vi "Data Read Single.vi"(0 "VISA resource name":refnum<visa-resource-name>, 5 "error in (no error)":errorcluster) -> (14 "VISA resource name out":refnum<visa-resource-name>, 15 "Measurement":dbl format="%#_6e", 19 "error out":errorcluster)   [LabVIEW 2024, in "Keithley 2100 Series.lvlib"]
doc: "This VI reads a measurement or calculation from the instrument. It also returns the channel number and units of the measurement (if applicable)."
uses:
  Keithley 2100 Series.lvlib
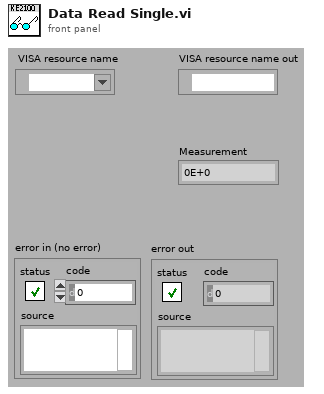
[diagram p1: front panel]
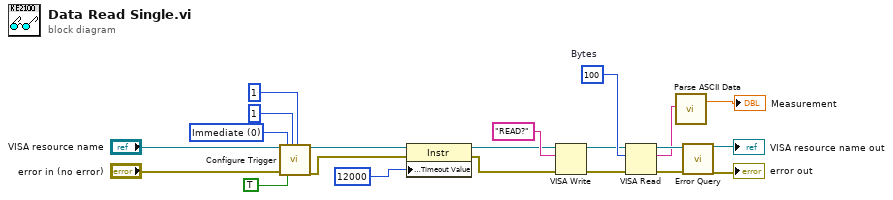
[diagram p0: block diagram]
diagram:
  w10 = u16 0 items=["Immediate", "Bus", "External"] ("Source (0: Immediate)")
  w21 = u32 100  # Bytes
  n1 = call "Configure Trigger.vi"("VISA resource name"="VISA resource name", "error in (no error)"="error in (no error)", "Source (0: Immediate)"=w10, "Auto Delay? (T: Auto)"=TRUE, "Sample Count (1)"=1, "Trigger Count (1)"=1 ("Sample Count (1)")) -> ("VISA resource name out"=w5:refnum<visa-resource-name>, "error out"=w4:errorcluster)  [unwired: 12 in]
  n2 = property class="Instr"(reference=w5, error in=w4, "General Settings:Timeout Value"=u32 12000) -> (reference out=w2:refnum<visa-resource-name>, error out=w3:errorcluster)
  n3 = VISA Write(VISA resource name=w2, write buffer="READ?", error in (no error)=w3) -> (VISA resource name out=w7:refnum<visa-resource-name>, error out=w6:errorcluster)  [unwired: 1 out]
  n4 = VISA Read(VISA resource name=w7, byte count=w21, error in (no error)=w6) -> (VISA resource name out=w20:refnum<visa-resource-name>, read buffer=w15:string, error out=w19:errorcluster)  [unwired: 1 out]
  n5 = call "Parse ASCII Data.vi"("ASCII Data (Empty)"=w15) -> ("Measurement"=→"Measurement":dbl)  [unwired: 18 in]
  n6 = call "Error Query.vi"("VISA resource name"=w20, "error in (no error)"=w19) -> ("VISA resource name out"=→"VISA resource name out":refnum<visa-resource-name>, "error out"=→"error out":errorcluster)  [unwired: 14 in, 2 out]
